vi "Channel Groups Page.vi"(8 "error in (no error)":errorcluster, 11 "Node Ptr":T1 format="%.0x") -> (0 "error out":errorcluster)   [LabVIEW 2027, in "Embedded Data Logger System Explorer.lvlib"]
uses:
  Embedded Data Logger System Explorer.lvlib
  <vilib>/NI VeriStand/Custom Device API/Custom Device Item Ref.ctl
  <vilib>/NI VeriStand/Custom Device API/Custom Device API.lvlib
  Scripting/Embedded Data Logger Scripting.lvlib
panel:
  in  "Channel Groups":i32(listbox)
  in  "Remove":bool
  in  "Add Channel Group":bool
  in  "Header":cluster{"Section Name":string}={"Section Name"="Log File Channel Groups"}
  out "Name":string
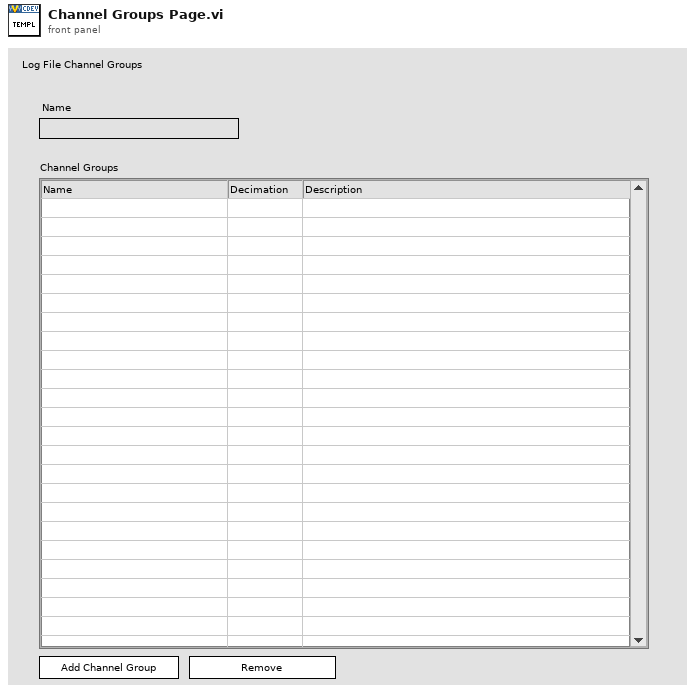
[diagram p1: front panel]
types:
  T1 = typedef "Custom Device API.lvlib/Custom Device Item Ref.ctl" = u64
  T2 = typedef "Custom Device API.lvlib/Custom Device Item Info.ctl" = cluster{"Name":string, "Is Channel":bool, "GUID":string, "Is Waveform":bool}
  T3 = typedef "Custom Device API.lvlib/Custom Device Commands.ctl" = enum16{"Default", "Item renamed", "Shutdown", "Dynamic button pressed"}
  T4 = typedef "LVRowAndColumnTypeDef.ctl" = cluster{"Row":i32, "Column":i32}
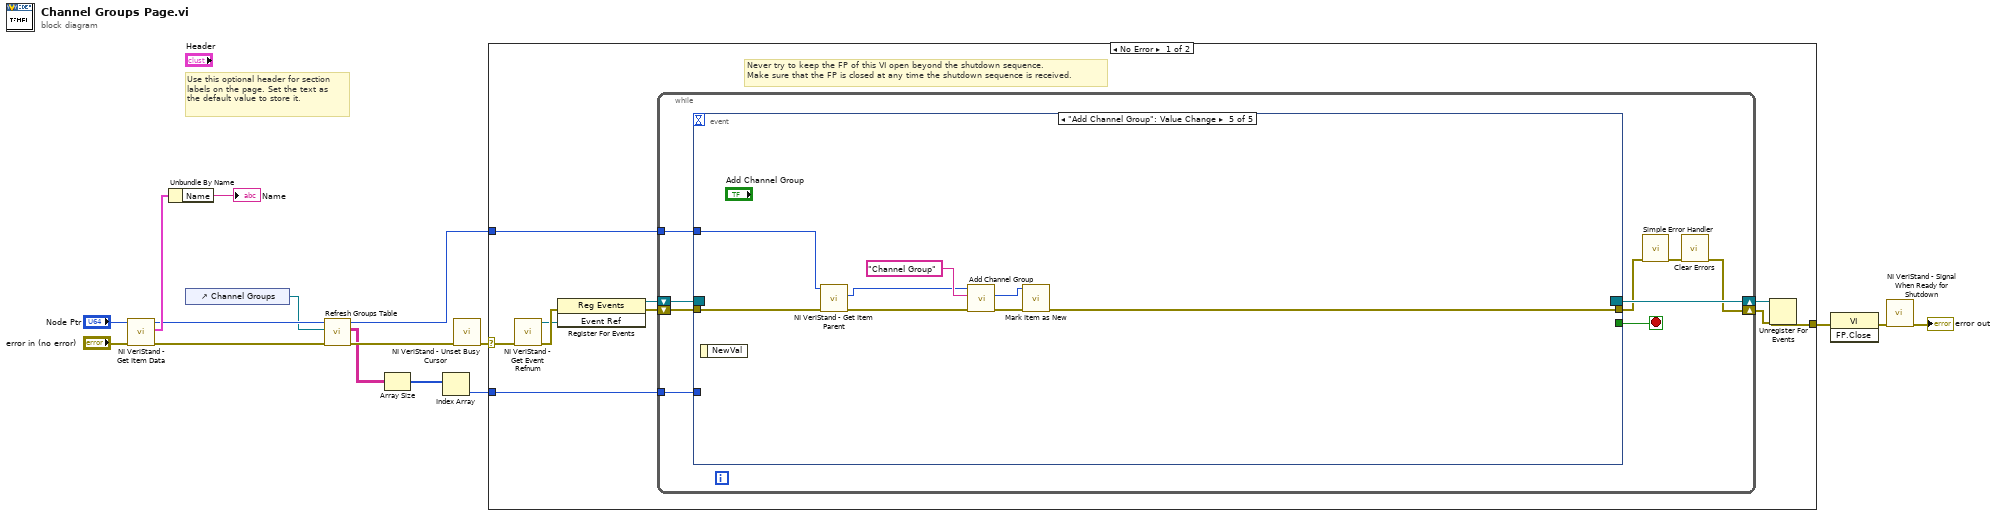
[diagram p0: block diagram]
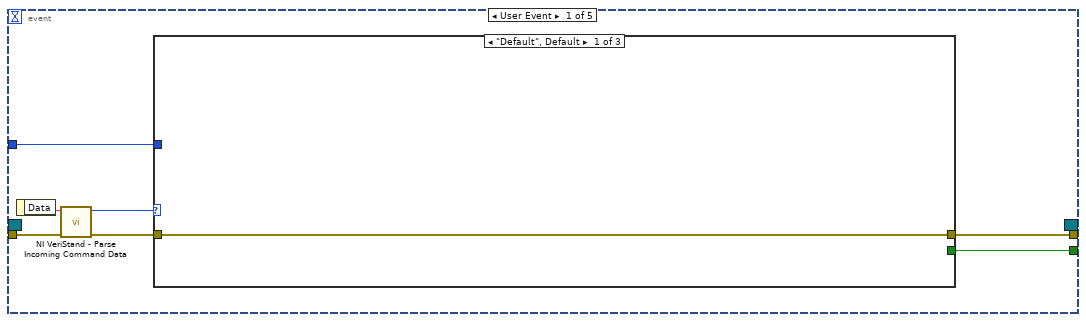
[diagram p2: hidden frame]
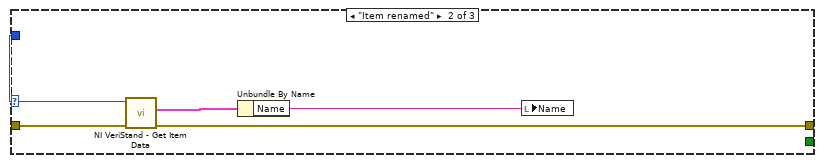
[diagram p3: hidden frame]
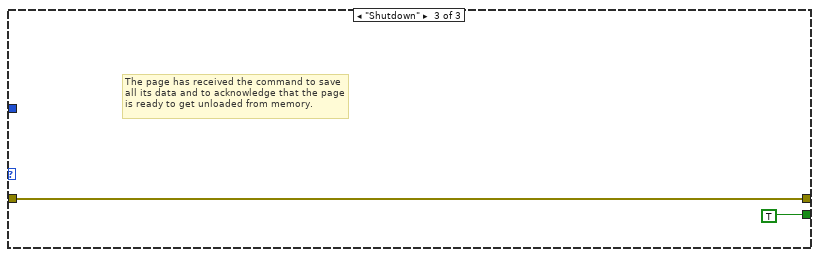
[diagram p4: hidden frame]
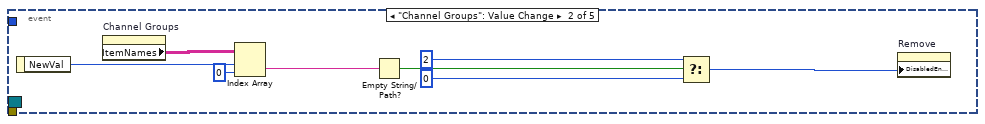
[diagram p5: hidden frame]
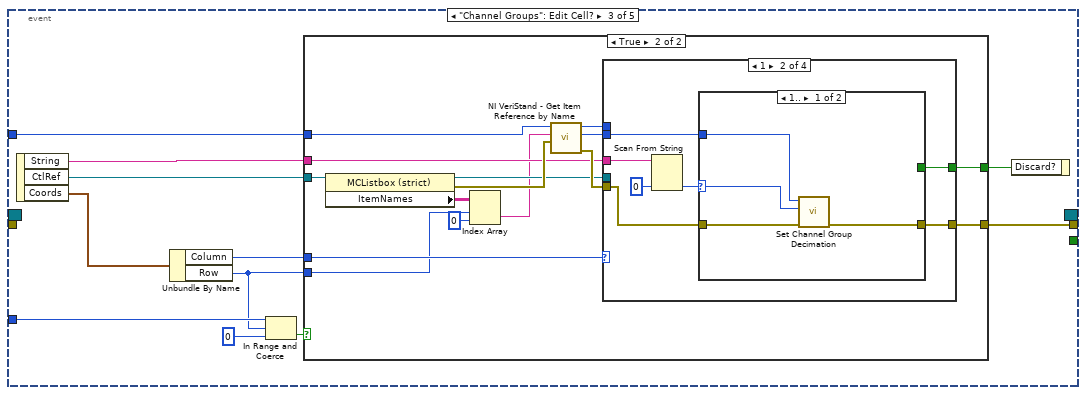
[diagram p6: hidden frame]
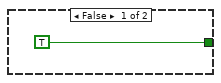
[diagram p7: hidden frame]
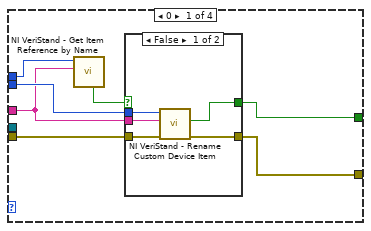
[diagram p8: hidden frame]
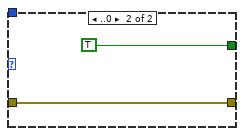
[diagram p10: hidden frame]
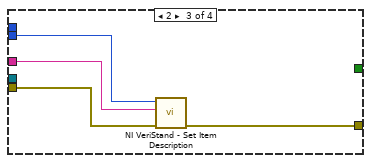
[diagram p11: hidden frame]
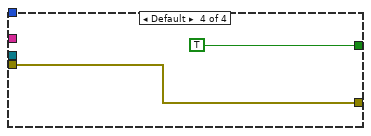
[diagram p12: hidden frame]
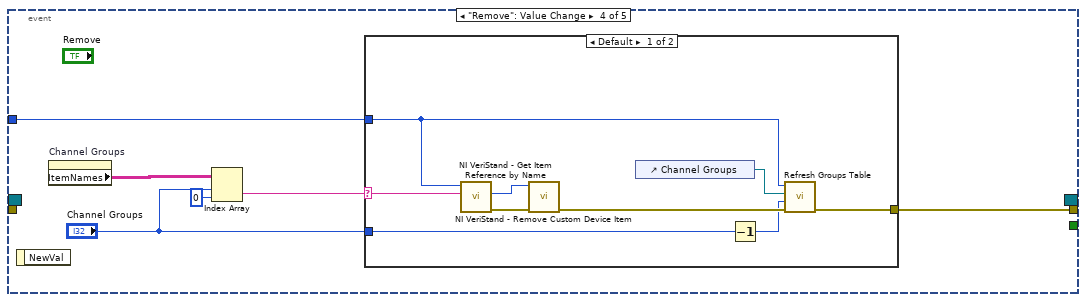
[diagram p13: hidden frame]
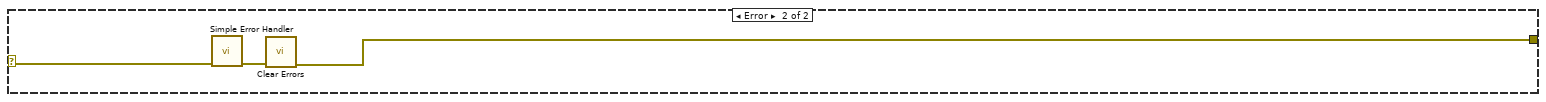
[diagram p15: hidden frame]
diagram:
  # "Use this optional header for section labels on the page. Set the text as the default value to store it."
  n1 = call <vilib>:"NI VeriStand - Get Item Data.vi"("error in (no error)"="error in (no error)", "Item Ref in"="Node Ptr") -> ("error out"=w8:errorcluster, "Item Info"=w10:T2, "Item Ref out"=w2:T1)  [unwired: 7 out]
  n2 = Unbundle By Name(w10) -> ("Name"=→"Name":string)
  n3 = control-ref of="Channel Groups"() -> (w1:refnum<vi>)
  n4 = call "Refresh Groups Table.vi"("error in (no error)"=w8, "MulticolumnListbox in"=w1, "Item Ref in"=w2) -> ("error out"=w6:errorcluster, "Array"=w5:string[][], "Item Ref out"=w7:T1)  [unwired: 6 in]
  n5 = Array Size(array=w5) -> (size(s)=w4:i32[])
  n6 = Index Array(array=w4) -> (element=w3:i32)  [unwired: 1 in]
  n7 = call <vilib>:"NI VeriStand - Unset Busy Cursor.vi"("error in (no error)"=w6) -> ("error out"=w12:errorcluster)  [unwired: 10 out]
  n8 = case shown="No Error" w12 {
    selector: w12 -> [w18 w144]
    tunnel: [w23 w142] -> w16
    tunnel: w7 -> [w19 _]
    tunnel: w3 -> [w17 _]
    frame No Error {
      # "Never try to keep the FP of this VI open beyond the shutdown sequence.\nMake sure that the FP is closed at any time the shutdown sequence is received."
      n9 = call <vilib>:"NI VeriStand - Get Event Refnum.vi"("error in (no error)"=w18) -> ("error out"=w26:errorcluster, "Event Ref"=w22:refnum<user-event>)  [unwired: 9 out]
      n10 = register-events(error in=w26, w22) -> (reference out=w20:refnum<event-registration>, error out=w21:errorcluster)  [unwired: 1 in]
      n11 = while {
        tunnel: w19 -> [w31]
        shift-right: [w28] -> w24
        shift-left: w21 -> [w34]
        shift-right: [w35] -> w25
        shift-left: w20 -> [w33]
        tunnel: w17 -> [w27]
        stop <- w32 stop-if-true
        n12 = event shown="[4] \"Add Channel Group\": Value Change" {
          selector: w33 -> [_ _ _ _ _]
          dyn-events: [_ _ _ _ _] -> w35
          timeout: _ -> [_ _ _ _ _]
          tunnel: w34 -> [w42 _ _ _ w141]
          tunnel: [w38 _ _ _ _] -> w32
          tunnel: [w37 _ w62 w120 w135] -> w30
          tunnel: w31 -> [w36 _ w66 w121 w137]
          tunnel: w27 -> [_ _ w65 _ _]
          event User Event {
            n13 = event-data() -> ("Data"=w41:string)  [unwired: 1 out]
            n14 = call <vilib>:"NI VeriStand - Parse Incoming Command Data.vi"("error in (no error)"=w42, "Incoming data"=w41) -> ("error out"=w40:errorcluster, "Action"=w39:T3)  [unwired: 8 out]
            n15 = case shown="\"Default\", Default" w39 {
              tunnel: w40 -> [w43 w48 w49]
              tunnel: [_ _ TRUE] -> w38
              tunnel: [w43 w45 w49] -> w37
              tunnel: w36 -> [_ w47 _]
              frame "Default", Default {
              }
              frame "Item renamed" {
                n16 = call <vilib>:"NI VeriStand - Get Item Data.vi"("error in (no error)"=w48, "Item Ref in"=w47) -> ("error out"=w45:errorcluster, "Item Info"=w46:T2)  [unwired: 8 out]
                n17 = Unbundle By Name(w46) -> ("Name"=w44:string)
                n18 = local write "Name"(w44) -> ()
              }
              frame "Shutdown" {
                # "The page has received the command to save all its data and to acknowledge that the page is ready to get unloaded from memory."
              }
            }
          }
          event "Channel Groups": Value Change {
            n19 = event-data() -> ("NewVal"=w52:i32)  [unwired: 1 out]
            n20 = property on="Channel Groups" class="MCListbox (strict)"() -> ("ItemNames"=w55:string[][])  [unwired: 2 in, 2 out]
            n21 = Index Array(array=w55, index (row)=w52, index (col)=0 ("disabled index (col)")) -> (element=w54:string)
            n22 = Empty String/Path?(string/path=w54) -> (empty?=w53:bool)
            n23 = Select(t=u8 2, s=w53, f=u8 0) -> (s? t:f=w56:u8)
            n24 = property on="Remove" class="Bool"("DisabledEnum"=w56) -> ()  [unwired: 2 in, 2 out]
          }
          event "Channel Groups": Edit Cell? {
            n25 = event-data() -> ("String"=w67:string, "CtlRef"=w59:refnum<vi>, "Coords"=w60:T4)  [unwired: 1 out]
            n26 = Unbundle By Name(w60) -> ("Column"=w69:i32, "Row"=w63:i32)
            n27 = In Range and Coerce(upper limit=w65, x=w63, lower limit=0) -> (In Range?=w61:bool)  [unwired: 1 out]
            n28 = case shown="True" w61 {
              tunnel: w59 -> [_ w83]
              tunnel: [TRUE w80] -> w68
              tunnel: w67 -> [_ w78]
              tunnel: w66 -> [_ w76]
              tunnel: w63 -> [_ w75]
              tunnel: w69 -> [_ w81]
              tunnel: [_ w77] -> w62
              frame False {
              }
              frame True {
                n29 = property class="MCListbox (strict)"(reference=w83) -> (reference out=w79:refnum<vi>, error out=w85:errorcluster, "ItemNames"=w82:string[][])  [unwired: 1 in]
                n30 = Index Array(array=w82, index (row)=w75, index (col)=0 ("disabled index (col)")) -> (element=w73:string)
                n31 = call <vilib>:"NI VeriStand - Get Item Reference by Name.vi"("error in (no error)"=w85, "Item Name"=w73, "Parent Ref in"=w76) -> ("error out"=w84:errorcluster, "Item Ref"=w72:T1, "Parent Ref out"=w71:T1)  [unwired: 5 in, 1 out]
                n32 = case shown="1" w81 {
                  tunnel: [w86 w102 _ TRUE] -> w80
                  tunnel: w72 -> [w91 w100 w115 _]
                  tunnel: w84 -> [w92 w104 w113 w117]
                  tunnel: w79 -> [_ _ _ _]
                  tunnel: w78 -> [w88 w106 w114 _]
                  tunnel: [w90 w101 w116 w117] -> w77
                  tunnel: w71 -> [w89 _ _ _]
                  frame 0 {
                    n33 = call <vilib>:"NI VeriStand - Get Item Reference by Name.vi"("Item Name"=w88, "Parent Ref in"=w89) -> ("Found"=w87:bool)  [unwired: 6 in, 3 out]
                    n34 = case shown="False" w87 {
                      selector: w87 -> [_ w98]
                      tunnel: w92 -> [w97 w99]
                      tunnel: w91 -> [w96 _]
                      tunnel: [w95 w99] -> w90
                      tunnel: w88 -> [w94 _]
                      tunnel: [w93 w98] -> w86
                      frame False {
                        n35 = call <vilib>:"NI VeriStand - Rename Custom Device Item.vi"("error in (no error)"=w97, "New Name"=w94, "Item Ref in"=w96) -> ("error out"=w95:errorcluster, "Request invalid?"=w93:bool)  [unwired: 6 in, 1 out]
                      }
                      frame True {
                        # "Ignore. Group\nby that name\nalready exists."
                      }
                    }
                  }
                  frame 1 {
                    n36 = Scan From String(input string=w106, default 1=0 ("default value 1")) -> (output 1=w103:i32)  [unwired: 3 in, 3 out]
                    n37 = case shown="1.." w103 {
                      selector: w103 -> [w107 _]
                      tunnel: w104 -> [w109 w111]
                      tunnel: [_ TRUE] -> w102
                      tunnel: [w108 w111] -> w101
                      tunnel: w100 -> [w110 _]
                      frame 1.. {
                        n38 = call "Set Channel Group Decimation.vi"("error in"=w109, "decimation"=w107, "channel group in"=w110) -> ("error out"=w108:errorcluster)  [unwired: 7 in, 1 out]
                      }
                      frame ..0 {
                      }
                    }
                  }
                  frame 2 {
                    n39 = call <vilib>:"NI VeriStand - Set Item Description.vi"("error in (no error)"=w113, "Description"=w114, "Item Ref in"=w115) -> ("error out"=w116:errorcluster)  [unwired: 6 in, 2 out]
                  }
                  frame Default {
                  }
                }
              }
            }
            n40 = event-data("Discard?"=w68) -> ()  [unwired: 1 in, 1 out]
          }
          event "Remove": Value Change {
            n41 = event-data() -> ()  [unwired: 2 out]
            n42 = property on="Channel Groups" class="MCListbox (strict)"() -> ("ItemNames"=w124:string[][])  [unwired: 2 in, 2 out]
            n43 = Index Array(array=w124, index (row)="Channel Groups", index (col)=0 ("disabled index (col)")) -> (element=w122:string)
            n44 = case shown="Default" w122 {
              selector: w122 -> [w132 _]
              tunnel: w121 -> [w127 _]
              tunnel: [w128 _] -> w120
              tunnel: "Channel Groups" -> [w126 _]
              frame Default {
                n45 = call <vilib>:"NI VeriStand - Get Item Reference by Name.vi"("Item Name"=w132, "Parent Ref in"=w127) -> ("error out"=w133:errorcluster, "Item Ref"=w131:T1)  [unwired: 6 in, 2 out]
                n46 = call <vilib>:"NI VeriStand - Remove Custom Device Item.vi"("error in (no error)"=w133, "Item Ref in"=w131) -> ("error out"=w129:errorcluster)  [unwired: 8 in, 1 out]
                n47 = control-ref of="Channel Groups"() -> (w130:refnum<vi>)
                n48 = Decrement(x=w126) -> (x-1=w125:i32)
                n49 = call "Refresh Groups Table.vi"("error in (no error)"=w129, "Index"=w125, "MulticolumnListbox in"=w130, "Item Ref in"=w127) -> ("error out"=w128:errorcluster)  [unwired: 5 in, 2 out]
              }
              frame "" {
              }
            }
          }
          event "Add Channel Group": Value Change {
            n50 = event-data() -> ()  [unwired: 2 out]
            n51 = call <vilib>:"NI VeriStand - Get Item Parent.vi"("error in (no error)"=w141, "Item Ref in"=w137) -> ("error out"=w138:errorcluster, "Parent Ref"=w136:T1)  [unwired: 6 in, 2 out]
            n52 = call "Add Channel Group.vi"("error in"=w138, "group name"="Channel Group" ("Name in"), "log file in"=w136) -> ("error out"=w140:errorcluster, "channel group"=w134:T1)  [unwired: 6 in, 1 out]
            n53 = call "Mark Item as New.vi"("error in (no error)"=w140, "Item Ref in"=w134) -> ("error out"=w135:errorcluster)  [unwired: 8 in, 1 out]
          }
        }
        n54 = call <vilib>:"Simple Error Handler.vi"("error in (no error)"=w30) -> ("error out"=w29:errorcluster)  [unwired: 1 in, 7 out]
        n55 = call <vilib>:"Clear Errors.vi"("error in (no error)"=w29) -> ("error out"=w28:errorcluster)  [unwired: 1 in, 5 out]
      }
      n56 = Unregister For Events(event registration refnum=w25, error in=w24) -> (error out=w23:errorcluster)
    }
    frame Error {
      n57 = call <vilib>:"Simple Error Handler.vi"("error in (no error)"=w144) -> ("error out"=w143:errorcluster)  [unwired: 1 in, 7 out]
      n58 = call <vilib>:"Clear Errors.vi"("error in (no error)"=w143) -> ("error out"=w142:errorcluster)  [unwired: 1 in, 5 out]
    }
  }
  n59 = invoke class="VI" method="FP.Close"(error in=w16) -> (error out=w15:errorcluster)  [unwired: 2 in, 2 out]
  n60 = call <vilib>:"NI VeriStand - Signal When Ready for Shutdown.vi"("error in (no error)"=w15) -> ("error out"=→"error out":errorcluster)  [unwired: 10 out]
